vi "Turn Degrees.vi"(2 "Tolerance":dbl, 3 "Degrees":dbl, 4 "Reset First?":bool) -> (0 "Motor Powers":cluster{"RMotor":dbl, "LMotor":dbl}, 1 "In Range?":bool)   [LabVIEW 2013]
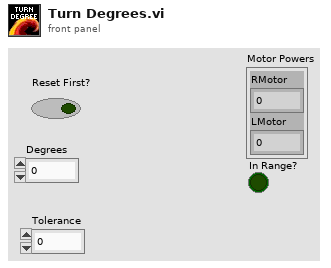
[diagram p1: front panel]
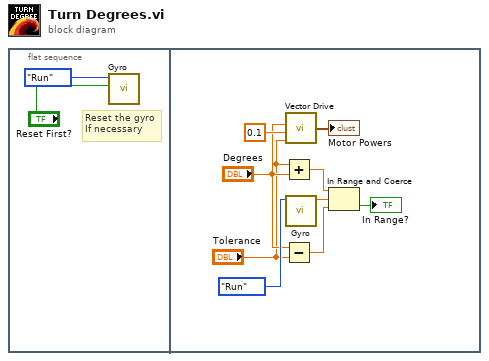
[diagram p0: block diagram]
diagram:
  n1 = flat-sequence {
    frame #0 {
      # "Reset the gyro\nIf necessary"
      n2 = call "Gyro.vi"("Reset"="Reset First?", "Enum"=enum16{"Start", "Run", "End"}."Run") -> ()  [unwired: 9 in, 1 out]
    }
    frame #1 {
      n3 = Add(x="Tolerance", y="Degrees") -> (x+y=w8:dbl)
      n4 = Subtract(x="Degrees", y="Tolerance") -> (x-y=w7:dbl)
      n5 = call "Vector Drive.vi"("Tolerance"="Tolerance", "Min. Power"=0.1, "Angle"="Degrees") -> ("Motor Powers"=→"Motor Powers":cluster{"RMotor":dbl, "LMotor":dbl})  [unwired: 1 in]
      n6 = call "Gyro.vi"("Enum"=enum16{"Start", "Run", "End"}."Run") -> ("Angle"=w11:dbl)  [unwired: 10 in]
      n7 = In Range and Coerce(upper limit=w8, x=w11, lower limit=w7) -> (In Range?=→"In Range?":bool)  [unwired: 1 out]
    }
  }
